vi "Store Tovey Data.vi"(8 "error in (no error)":errorcluster, 11 "Model in":refnum<class "Model.lvclass">) -> (0 "error out":errorcluster, 3 "Model out":refnum<class "Model.lvclass">)   [LabVIEW 2016]
uses:
  Model.lvclass
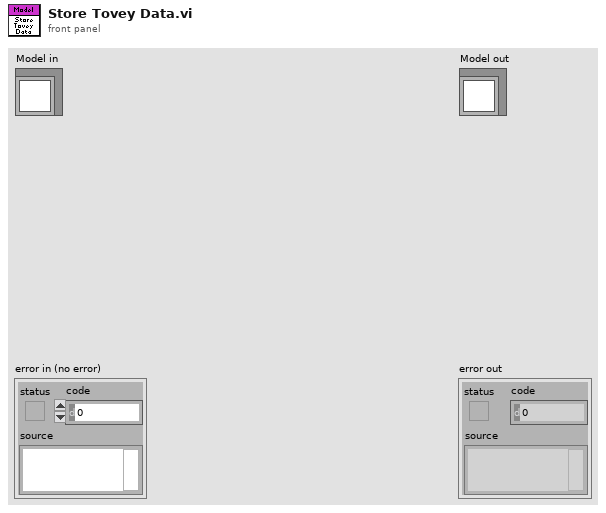
[diagram p1: front panel]
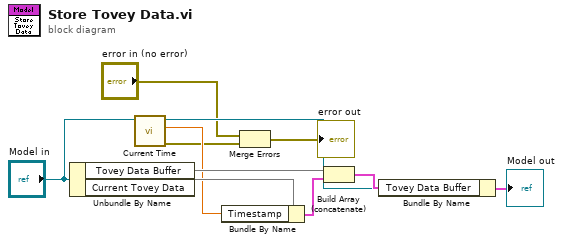
[diagram p0: block diagram]
diagram:
  n1 = Unbundle By Name("Model in") -> ("Tovey Data Buffer"=w11, "Current Tovey Data"=w8)
  n2 = call "Current Time.vi"("Model in"="Model in") -> ("error out"=w3:errorcluster, "Time"=w4:dbl, "Model out"=w5:refnum<class "Model.lvclass">)  [unwired: 8 in]
  n3 = Bundle By Name(cluster=w8, "Timestamp"=w4) -> (w7:cluster{})
  n4 = Merge Errors("error in (no error)", w3) -> (→"error out":errorcluster)
  n5 = Build Array (concatenate)(w11, w7) -> (w10:cluster{}[])
  n6 = Bundle By Name(cluster=w5, "Tovey Data Buffer"=w10) -> (→"Model out":cluster{})
